vi "Initialize.vi"(8 "error in (no error)":errorcluster, 11 "S4ACS_GUI in":refnum<class "GuiderSetup.lvclass">) -> (0 "error out":errorcluster, 3 "S4ACS_GUI out":refnum<class "GuiderSetup.lvclass">)   [LabVIEW 2018, in "GuiderSetup.lvclass"]
uses:
  GuiderSetup.lvclass
  C:/Users/devstaff/sparc4/s4gui/Versao ZeroMQ REQ-REP/SPARC4_GUI -v1.0.0/S4GUI/S4GUI.lvclass
  S4GUI/S4GUI.lvclass/S4GUI.ctl
  GuiderSetup.lvclass/GuiderSetup.ctl
  Instrument/Instrument.lvclass
  PublisherGS/PublisherGS.lvclass
  AG/AG.lvclass
  S4GUI/S4GUI.lvclass
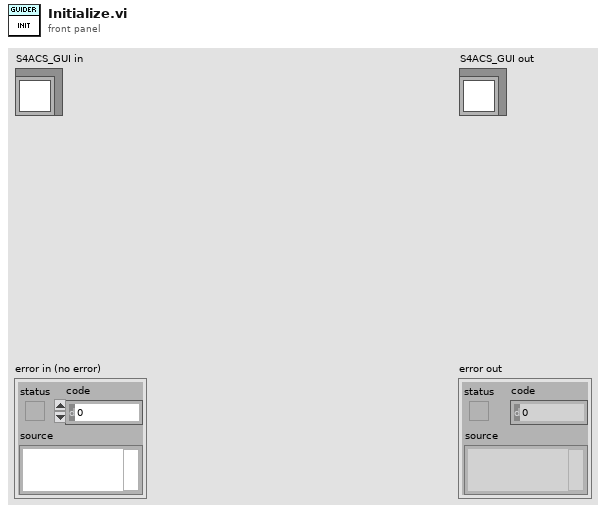
[diagram p1: front panel]
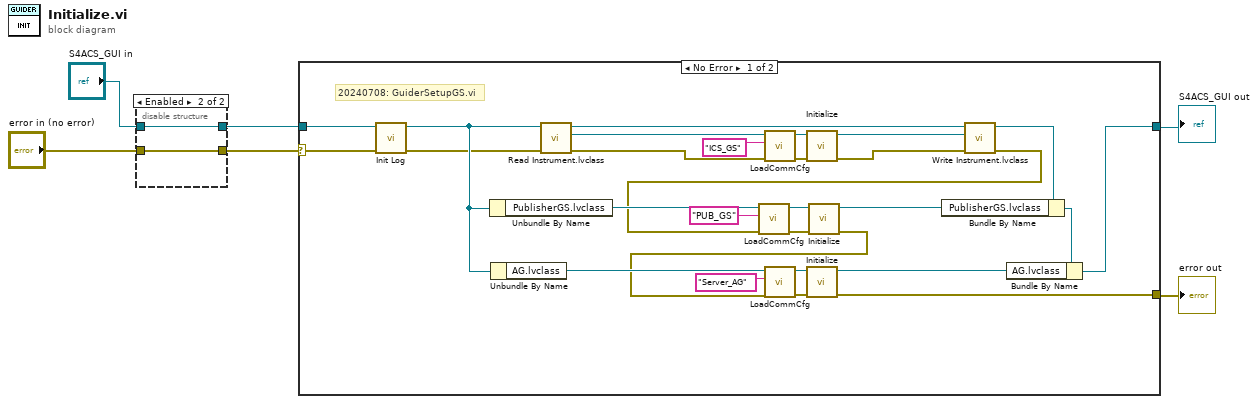
[diagram p0: block diagram]
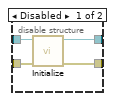
[diagram p2: hidden frame]
diagram:
  n1 = disable-structure shown="Enabled" {
    disable-tunnel: "error in (no error)" -> [w10 w11]
    disable-tunnel: "S4ACS_GUI in" -> [w9 w12]
    disable-tunnel: [w8 w12] -> w4
    disable-tunnel: [w7 w11] -> w3
    frame Disabled {
      n2 = call-parent "Initialize.vi"("error in (no error)"=w10, "S4ACS_GUI in"=w9) -> ("error out"=w7:errorcluster, "S4ACS_GUI out"=w8:refnum<class "GuiderSetup.lvclass">)  [unwired: 8 in]
    }
    frame Enabled {
    }
  }
  n3 = case shown="No Error" w3 {
    selector: w3 -> [w15 w41]
    tunnel: w4 -> [w16 w42]
    tunnel: [w24 w41] -> w1
    tunnel: [w39 w42] -> w2
    frame No Error {
      # "20240708: GuiderSetupGS.vi"
      n4 = call-dynamic "Init Log.vi"("error in (no error)"=w15, "GuiderSetup in"=w16) -> ("error out"=w13:errorcluster, "GuiderSetup out"=w14:refnum<class "GuiderSetup.lvclass">)  [unwired: 8 in]
      n5 = Unbundle By Name(w14) -> ("PublisherGS.lvclass"=w20:refnum<class "PublisherGS.lvclass">)
      n6 = Unbundle By Name(w14) -> ("AG.lvclass"=w34:refnum<class "AG.lvclass">)
      n7 = call "Read Instrument.lvclass.vi"("error in (no error)"=w13, "S4ACS_GUI in"=w14) -> ("error out"=w37:errorcluster, "Instrument.lvclass"=w38:refnum<class "Instrument.lvclass">, "S4ACS_GUI out"=w28:refnum<class "GuiderSetup.lvclass">)  [unwired: 7 in]
      n8 = call-dynamic "LoadCommCfg.vi"("error in (no error)"=w37, "section (server name)"="ICS_GS", "Server in"=w38) -> ("error out"=w36:errorcluster, "Server out"=w35:refnum<class "Instrument.lvclass">)  [unwired: 7 in]
      n9 = call-dynamic "Initialize.vi"("error in (no error)"=w36, "Instrument in"=w35) -> ("error out"=w27:errorcluster, "Instrument out"=w29:refnum<class "Instrument.lvclass">)  [unwired: 8 in]
      n10 = call "Write Instrument.lvclass.vi"("error in (no error)"=w27, "Instrument.lvclass"=w29, "S4ACS_GUI in"=w28) -> ("error out"=w18:errorcluster, "S4ACS_GUI out"=w22:refnum<class "GuiderSetup.lvclass">)  [unwired: 7 in]
      n11 = call-dynamic "LoadCommCfg.vi"("error in (no error)"=w18, "section (server name)"="PUB_GS", "Client in"=w20) -> ("error out"=w25:errorcluster, "Client out"=w23:refnum<class "PublisherGS.lvclass">)  [unwired: 7 in]
      n12 = call-dynamic "Initialize.vi"("error in (no error)"=w25, "Client in"=w23) -> ("error out"=w17:errorcluster, "Client out"=w19:refnum<class "PublisherGS.lvclass">)  [unwired: 8 in]
      n13 = call-dynamic "LoadCommCfg.vi"("error in (no error)"=w17, "section (server name)"="Server_AG", "Client in"=w34) -> ("error out"=w32:errorcluster, "Client out"=w33:refnum<class "AG.lvclass">)  [unwired: 7 in]
      n14 = call-dynamic "Initialize.vi"("error in (no error)"=w32, "AG in"=w33) -> ("error out"=w24:errorcluster, "AG out"=w40:refnum<class "AG.lvclass">)  [unwired: 8 in]
      n15 = Bundle By Name(cluster=w22, "PublisherGS.lvclass"=w19) -> (w21:refnum<class "GuiderSetup.lvclass">)
      n16 = Bundle By Name(cluster=w21, "AG.lvclass"=w40) -> (w39:refnum<class "GuiderSetup.lvclass">)
    }
    frame Error {
    }
  }
  "error out" <- w1
  "S4ACS_GUI out" <- w2
